vi "TCP-Generic Listener.vi"(5 "port":u16, 11 "error in (no error)":errorcluster) -> (4 "connection ID":refnum<k5>, 8 "Connected?":bool, 15 "error out":errorcluster)   [LabVIEW 2020]
panel:
  in  "net address":u32
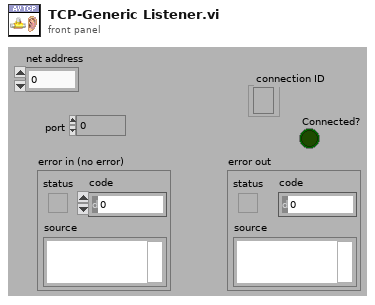
[diagram p1: front panel]
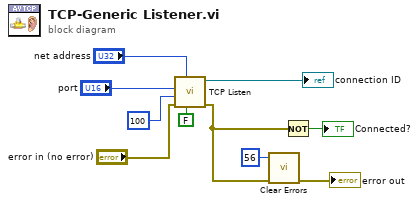
[diagram p0: block diagram]
diagram:
  n1 = call <vilib>:"TCP Listen.vi"("resolve remote address (T)"=FALSE, "net address"="net address", "error in (no error)"="error in (no error)", "timeout ms (wait forever: -1)"=100, "port"="port") -> ("error out"=w3:errorcluster, "connection ID"=→"connection ID":refnum<k5>)  [unwired: 2 in, 3 out]
  n2 = call <vilib>:"Clear Errors.vi"("error in (no error)"=w3, "specific error code to clear (0: all)"=56) -> ("error out"=→"error out":errorcluster)  [unwired: 4 in, 1 out]
  n3 = Not(x=w3) -> (.not. x?=→"Connected?":bool)
